vi "Save data.vi"(7 "file path (use dialog)":path=path "/home/lvuser/natinst/bin/DaNIdata.txt", 8 "Obsticle map":u16[][](array[ring]), 9 "Robot angle":dbl, 10 "Actual robot location":dbl[](array[numeric]), 11 "Map dimensions":dbl[](array[numeric])) -> ()   [LabVIEW 2015]
panel:
  out "first array":dbl[][](array[numeric])
  in  "format string":string
  out "text":string
  out "Data to be sent":dbl[][](array[numeric])
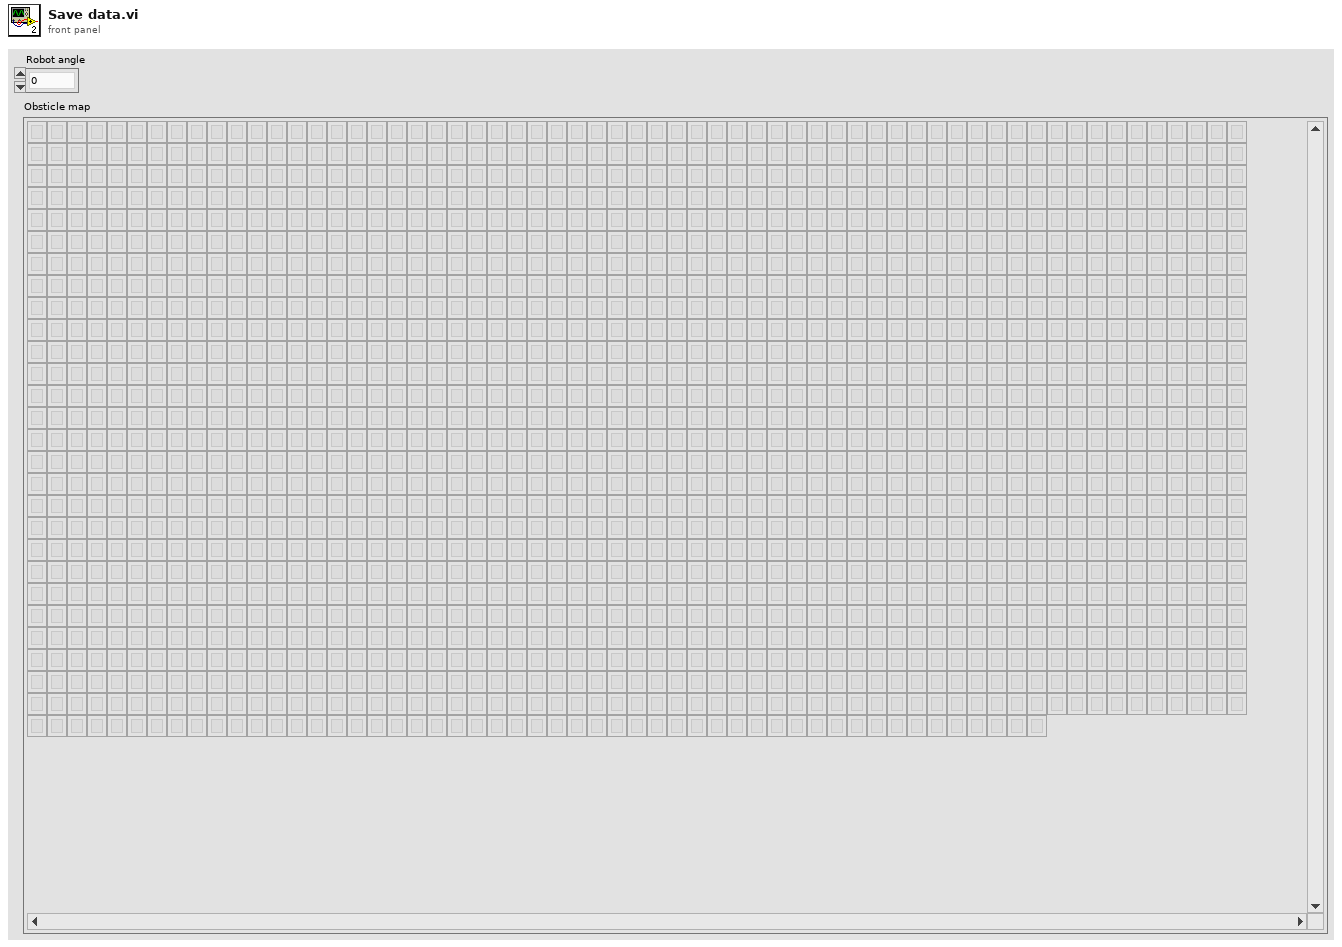
[diagram p1: front panel]
types:
  T1 = enum16{"open", "replace", "create", "open or create", "replace or create", "replace or create with confirmation"}
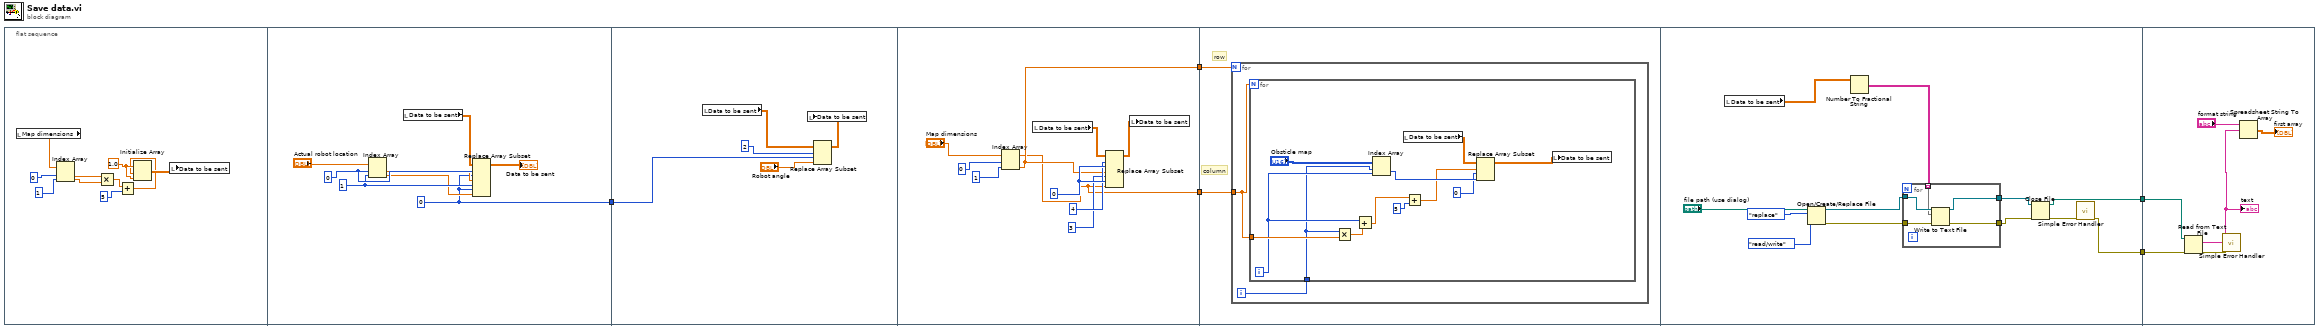
[diagram p0: block diagram]
diagram:
  n1 = flat-sequence {
    tunnel: [w16] -> w5
    tunnel: w5 -> [w25]
    tunnel: [w30] -> w4
    tunnel: [w29] -> w3
    tunnel: w4 -> [w40]
    tunnel: w3 -> [w39]
    tunnel: [w56] -> w2
    tunnel: [w55] -> w1
    tunnel: w2 -> [w73]
    tunnel: w1 -> [w72]
    frame #0 {
      w9 = 1.0
      n2 = local read "Map dimensions"() -> (w14:dbl[])
      n3 = Index Array(array=w14, index #1=0, index #2=1) -> (element #1=w11:dbl, element #2=w10:dbl)
      n4 = Multiply(x=w11, y=w10) -> (x*y=w8:dbl)
      n5 = Add(x=w8, y=5) -> (x+y=w7:dbl)
      n6 = Initialize Array(w9, w7, w9) -> (w15:dbl[][])
      n7 = local write "Data to be sent"(w15) -> ()
    }
    frame #1 {
      w16 = 0
      w19 = 1
      w20 = 0
      n8 = Index Array(array="Actual robot location", index #1=w20, index #2=w19) -> (element #1=w18:dbl, element #2=w17:dbl)
      n9 = local read "Data to be sent"() -> (w22:dbl[][])
      n10 = Replace Array Subset(array=w22, new element #1=w18, index (row) #1=w20, index (col) #1=w16, new element #2=w17, index (row) #2=w19, index (col) #2=w16) -> (→"Data to be sent":dbl[][])
    }
    frame #2 {
      n11 = local read "Data to be sent"() -> (w28:dbl[][])
      n12 = Replace Array Subset(array=w28, new element="Robot angle", index (row)=2, index (col)=w25) -> (w27:dbl[][])
      n13 = local write "Data to be sent"(w27) -> ()
    }
    frame #3 {
      w36 = 0
      n14 = Index Array(array="Map dimensions", index #1=0, index #2=1) -> (element #1=w29:dbl, element #2=w30:dbl)
      n15 = local read "Data to be sent"() -> (w34:dbl[][])
      n16 = Replace Array Subset(array=w34, new element #1=w30, index (row) #1=4, index (col) #1=w36, new element #2=w29, index (row) #2=3, index (col) #2=w36) -> (w33:dbl[][])
      n17 = local write "Data to be sent"(w33) -> ()
    }
    frame #4 {
      # "row"
      # "column"
      n18 = for {
        N: w40 -> [_]
        tunnel: w39 -> [w41]
        i -> [w42]
        n19 = for {
          N: w41 -> [_]
          tunnel: w42 -> [w43]
          tunnel: w41 -> [w45]
          i -> [w44]
          n20 = Multiply(x=w43, y=w45) -> (x*y=w47:dbl)
          n21 = Add(x=w44, y=w47) -> (x+y=w46:dbl)
          n22 = Index Array(array="Obsticle map", index (row)=w43, index (col)=w44) -> (element=w51:u16)
          n23 = local read "Data to be sent"() -> (w52:dbl[][])
          n24 = Add(x=w46, y=5) -> (x+y=w48:dbl)
          n25 = Replace Array Subset(array=w52, new element=w51, index (row)=w48, index (col)=0) -> (w53:dbl[][])
          n26 = local write "Data to be sent"(w53) -> ()
        }
      }
    }
    frame #5 {
      n27 = local read "Data to be sent"() -> (w59:dbl[][])
      n28 = Open/Create/Replace File(file path (use dialog)="file path (use dialog)", operation (0:open)=T1."replace", access (0:read/write)=enum16{"read/write", "read-only", "write-only"}."read/write") -> (refnum out=w62:refnum<file>, error out=w63:errorcluster)  [unwired: 3 in, 1 out]
      n29 = Number To Fractional String(number=w59) -> (F-format string=w58:string[][])  [unwired: 3 in]
      n30 = for {
        tunnel: w62 -> [w71]
        tunnel: w63 -> [w70]
        tunnel: [w69] -> w60
        tunnel: [w68] -> w61
        tunnel: w58 -> [w67] mode=indexing
        n31 = Write to Text File(file (use dialog)=w71, text=w67, error in=w70) -> (refnum out=w69:refnum<file>, error out=w68:errorcluster)  [unwired: 1 in, 1 out]
      }
      n32 = Close File(refnum=w60, error in=w61) -> (path=w55:path, error out=w57:errorcluster)
      n33 = call <vilib>:"Simple Error Handler.vi"("error in (no error)"=w57) -> ("error out"=w56:errorcluster)  [unwired: 4 in, 4 out]
    }
    frame #6 {
      n34 = Read from Text File(file (use dialog)=w72, error in=w73) -> (text=w76:string, error out=w77:errorcluster)  [unwired: 2 in, 2 out]
      "text" <- w76
      n35 = call <vilib>:"Simple Error Handler.vi"("error in (no error)"=w77) -> ()  [unwired: 4 in, 5 out]
      n36 = Spreadsheet String To Array(format string="format string", spreadsheet string=w76) -> (array=→"first array":dbl[][])  [unwired: 2 in]
    }
  }
